vi "Rebuild Command Table.vi"   [LabVIEW 2019, in "LINXx.lvlib"]
doc: "Dev helper to automatically generate table of command codes from the base LinxListener code"
uses:
  LINXx.lvlib
  <vilib>/regexp/Match Regular Expression.xnode
types:
  T1 = enum16{"Native", "Native Command Line", "UNIX", "Macintosh", "DOS"}
  T2 = enum16{"open", "replace", "create", "open or create", "replace or create", "replace or create with confirmation"}
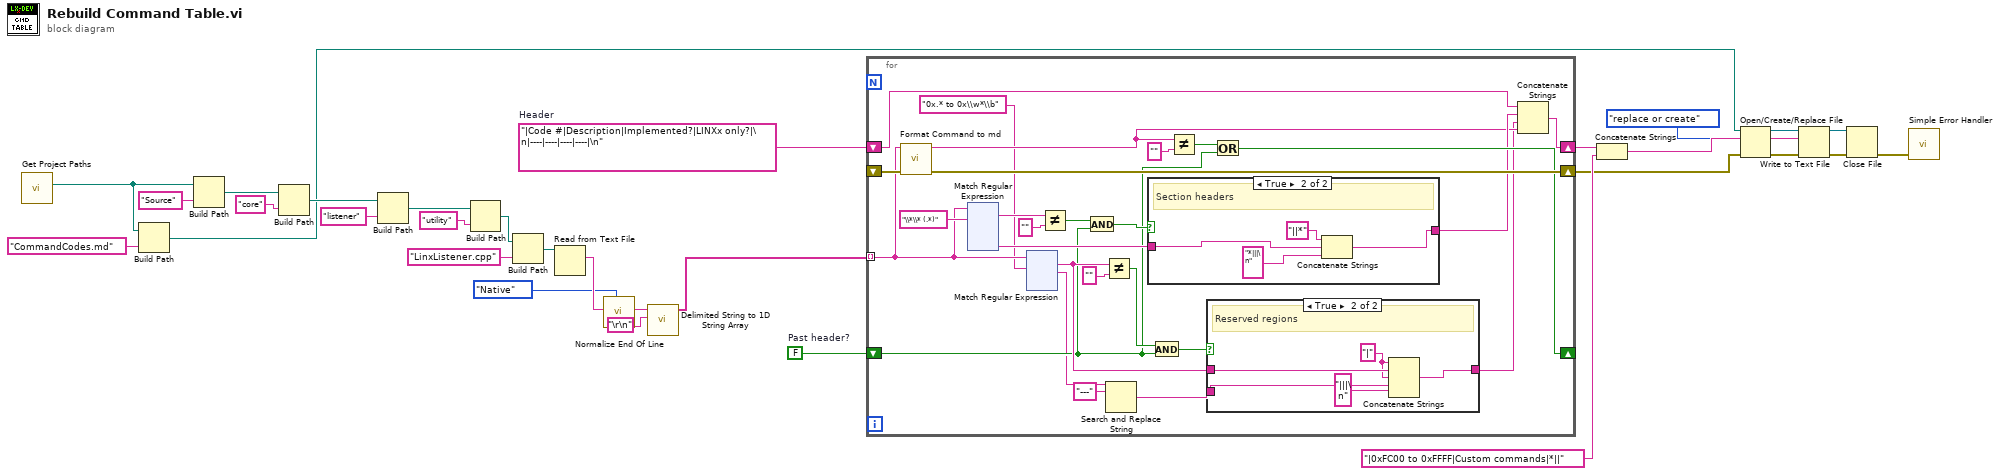
[diagram p0: block diagram]
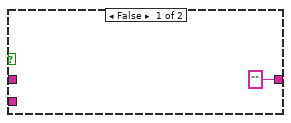
[diagram p2: hidden frame]
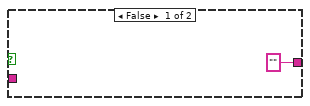
[diagram p3: hidden frame]
diagram:
  w17 = FALSE  # Past header?
  w18 = "|Code #|Description|Implemented?|LINXx only?|\n|----|----|----|----|\n"  # Header
  n1 = call "Get Project Paths.vi"() -> ("Firmware path"=w19:path)  [unwired: 9 in, 2 out]
  n2 = Build Path(base path=w19, name or relative path="CommandCodes.md") -> (appended path=w8:path)
  n3 = Build Path(base path=w19, name or relative path="Source") -> (appended path=w28:path)
  n4 = Build Path(base path=w28, name or relative path="core") -> (appended path=w26:path)
  n5 = Build Path(base path=w26, name or relative path="listener") -> (appended path=w24:path)
  n6 = Build Path(base path=w24, name or relative path="utility") -> (appended path=w22:path)
  n7 = Build Path(base path=w22, name or relative path="LinxListener.cpp") -> (appended path=w21:path)
  n8 = Read from Text File(file (use dialog)=w21) -> (text=w5:string)  [unwired: 3 in, 3 out]
  n9 = call <vilib>:"Normalize End Of Line.vi"("end of line (Native)"=T1."Native", "string in"=w5) -> ("string out"=w3:string)  [unwired: 6 in]
  n10 = call <vilib>:"Delimited String to 1D String Array.vi"("delimiter"="\r\n", "delimited string"=w3) -> ("string array"=w4:string[])  [unwired: 9 in]
  n11 = for {
    tunnel: w4 -> [w41] mode=indexing
    shift-right: [w55] -> w14
    shift-left: w18 -> [w56]
    shift-right: [w53] -> w9
    shift-left: _ -> [w54]
    shift-right: [w44] -> _
    shift-left: w17 -> [w34]
    n12 = call "Format Command to md.vi"("error in (no error)"=w54, "line"=w41) -> ("error out"=w53:errorcluster, ".md table row"=w42:string)  [unwired: 7 in, 1 out]
    n13 = xnode "Match Regular Expression"("input string"=w41, "regular expression"="\\*\\* (.*)") -> ("whole match"=w51:string, "submatch 1"=w48:string)  [unwired: 4 in, 4 out]
    n14 = xnode "Match Regular Expression"("input string"=w41, "regular expression"="0x.* to 0x\\w*\\b") -> ("whole match"=w35:string, "after match"=w32:string)  [unwired: 4 in, 3 out]
    n15 = Not Equal?(x=w51, y="") -> (x != y?=w49:bool)
    n16 = And(x=w49, y=w34) -> (x .and. y?=w47:bool)
    n17 = Not Equal?(x=w35, y="") -> (x != y?=w38:bool)
    n18 = Search and Replace String(input string=w32, search string="---") -> (result string=w33:string)  [unwired: 6 in, 3 out]
    n19 = case shown="True" w47 {
      tunnel: w48 -> [_ w180]
      tunnel: ["" w179] -> w43
      frame False {
      }
      frame True {
        # "Section headers"
        n20 = Concatenate Strings("||*" ("string"), w180, "*|||\n" ("string")) -> (w179:string)
      }
    }
    n21 = And(x=w38, y=w34) -> (x .and. y?=w39:bool)
    n22 = Not Equal?(x=w42, y="") -> (x != y?=w45:bool)
    n23 = case shown="True" w39 {
      tunnel: w35 -> [_ w62]
      tunnel: ["" w61] -> w36
      tunnel: w33 -> [_ w59]
      frame False {
      }
      frame True {
        w60 = "|" ("string")
        # "Reserved regions"
        n24 = Concatenate Strings(w60, w62, w60, w59, "|||\n" ("string")) -> (w61:string)
      }
    }
    n25 = Or(x=w45, y=w34) -> (x .or. y?=w44:bool)
    n26 = Concatenate Strings(w56, w43, w36, w42) -> (w55:string)
  }
  n27 = Concatenate Strings(w14, "|0xFC00 to 0xFFFF|Custom commands|*||" ("string")) -> (w13:string)
  n28 = Open/Create/Replace File(file path (use dialog)=w8, error in=w9, operation (0:open)=T2."replace or create") -> (refnum out=w11:refnum<file>, error out=w12:errorcluster)  [unwired: 3 in, 1 out]
  n29 = Write to Text File(file (use dialog)=w11, text=w13, error in=w12) -> (refnum out=w10:refnum<file>, error out=w16:errorcluster)  [unwired: 1 in, 1 out]
  n30 = Close File(refnum=w10, error in=w16) -> (error out=w6:errorcluster)  [unwired: 1 out]
  n31 = call <vilib>:"Simple Error Handler.vi"("error in (no error)"=w6) -> ()  [unwired: 4 in, 5 out]
